vi "TDTRX6-Load Signal Bank.vi"(1 "Action":T1=enum."Write", 7 "Output array":dbl[][](array[numeric]) format="%.2f", 11 "error in (no error)":errorcluster) -> (15 "error out":errorcluster={"status"=FALSE, "code"=0, "source"="."})   [LabVIEW 2015]
uses:
  TDT-Signal Bank Action.ctl
  TDT-Globals.vi
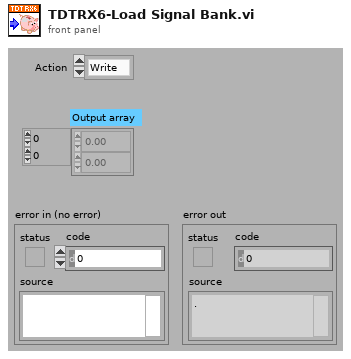
[diagram p1: front panel]
types:
  T1 = typedef "TDT-Signal Bank Action.ctl" = enum16{"Init", "Write", "Read", "Rewrite", "Reset", "Recycle", "Ramp up", "Ramp down", "Zero"}
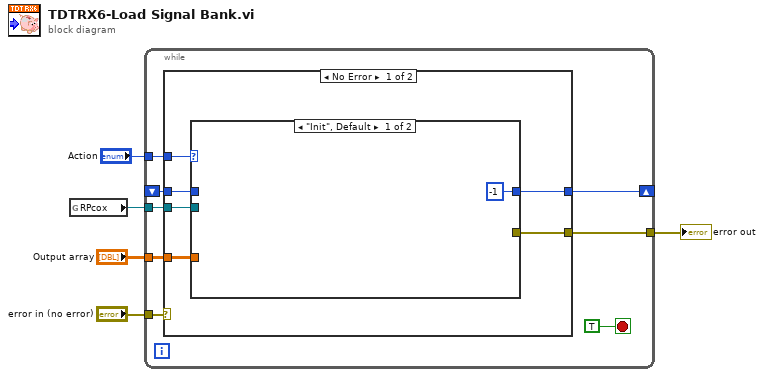
[diagram p0: block diagram]
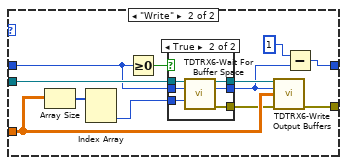
[diagram p2: hidden frame]
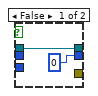
[diagram p3: hidden frame]
diagram:
  n1 = global read "TDT-Globals.vi" "RPcox"() -> (w3:refnum<k7>)
  n2 = while {
    tunnel: [w13] -> w5
    tunnel: "error in (no error)" -> [w12]
    tunnel: w3 -> [w11]
    tunnel: "Output array" -> [w10]
    tunnel: "Action" -> [w9]
    shift-right: [w7] -> _
    shift-left: _ -> [w6]
    stop <- TRUE stop-if-true
    n3 = case shown="No Error" w12 {
      selector: w12 -> [_ w42]
      tunnel: [w14 w42] -> w13
      tunnel: w11 -> [w15 _]
      tunnel: w10 -> [w19 _]
      tunnel: w9 -> [w18 _]
      tunnel: [w17 w41] -> w7
      tunnel: w6 -> [w16 w41]
      frame No Error {
        n4 = case shown="\"Init\", Default" w18 {
          tunnel: w19 -> [_ w29]
          tunnel: [-1 w31] -> w17
          tunnel: w16 -> [_ w22]
          tunnel: w15 -> [_ w27]
          tunnel: [_ w25] -> w14
          frame "Init", Default {
          }
          frame "Write" {
            n5 = Array Size(array=w29) -> (size(s)=w32:i32[])
            n6 = Index Array(array=w32) -> (element #2=w24:i32)  [unwired: 2 in, 1 out]
            n7 = Greater Or Equal To 0?(x=w22) -> (x >= 0?=w21:bool)
            n8 = case shown="True" w21 {
              tunnel: [_ w40] -> w28
              tunnel: w27 -> [w34 w39]
              tunnel: [w34 w38] -> w26
              tunnel: w22 -> [_ w37]
              tunnel: w24 -> [_ w36]
              tunnel: [0 ("Next Buffer Out") w35] -> w23
              frame False {
              }
              frame True {
                n9 = call "TDTRX6-Wait For Buffer Space.vi"("RPcox"=w39, "Next Buffer"=w37, "Buffer Length"=w36) -> ("RPcox Out"=w38:refnum<k7>, "Next Buffer Out"=w35:i32, "error out"=w40:errorcluster)  [unwired: 10 in]
              }
            }
            n10 = call "TDTRX6-Write Output Buffers.vi"("RPcox"=w26, "Next Buffer"=w23, "Input array"=w29, "error in (no error)"=w28) -> ("error out"=w25:errorcluster)  [unwired: 11 in]
            n11 = Subtract(x=1, y=w23) -> (x-y=w31:i32)
          }
        }
      }
      frame Error {
      }
    }
  }
  "error out" <- w5
